vi "DataGridView Specific Column DEMO.vi"() -> ()   [LabVIEW 2011]
uses:
  System.Windows.Forms
panel:
  in  "stop":bool
  in  "DataGridView":refnum<k24>(container)
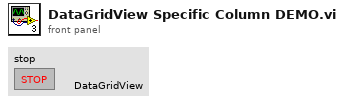
[diagram p1: front panel]
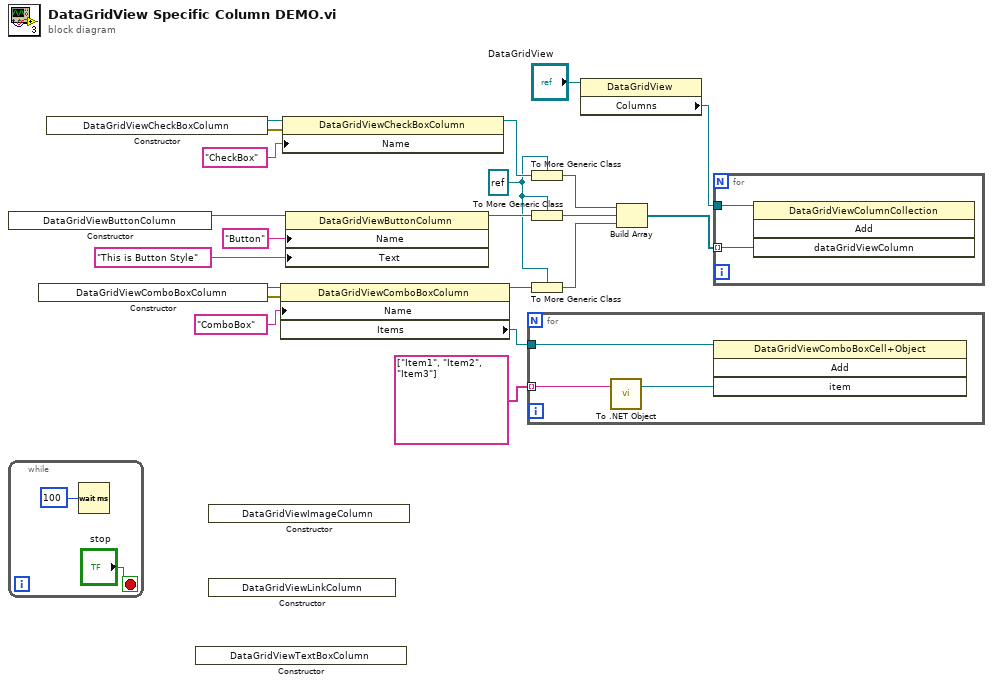
[diagram p0: block diagram]
diagram:
  w2 = refnum<k24> refnum ("dataGridViewColumn")
  n1 = constructor class="DataGridViewButtonColumn"() -> (reference out=w16:refnum<k24>)  [unwired: 3 in, 2 out]
  n2 = while {
    stop <- "stop" stop-if-true
    n3 = Wait (ms)(milliseconds to wait=u32 100) -> ()  [unwired: 1 out]
  }
  n4 = constructor class="DataGridViewComboBoxColumn"() -> (reference out=w7:refnum<k24>, error out=w8:errorcluster)  [unwired: 3 in, 1 out]
  n5 = constructor class="DataGridViewCheckBoxColumn"() -> (reference out=w20:refnum<k24>, error out=w19:errorcluster)  [unwired: 3 in, 1 out]
  n6 = constructor class="DataGridViewTextBoxColumn"() -> ()  [unwired: 3 in, 3 out]
  n7 = constructor class="DataGridViewImageColumn"() -> ()  [unwired: 3 in, 3 out]
  n8 = constructor class="DataGridViewLinkColumn"() -> ()  [unwired: 3 in, 3 out]
  n9 = property class="DataGridViewComboBoxColumn"(reference=w7, error in=w8, "Name"="ComboBox") -> (reference out=w3:refnum<k24>, "Items"=w4:refnum<k24>)  [unwired: 1 out]
  n10 = property class="DataGridViewCheckBoxColumn"(reference=w20, error in=w19, "Name"="CheckBox") -> (reference out=w13:refnum<k24>)  [unwired: 1 out]
  n11 = property class="DataGridViewButtonColumn"(reference=w16, "Name"="Button", "Text"="This is Button Style") -> (reference out=w12:refnum<k24>)  [unwired: 1 in, 1 out]
  n12 = for {
    tunnel: string[] ["Item1", "Item2", "Item3"] -> [w26] mode=indexing
    tunnel: w4 -> [w24]
    n13 = call <vilib>:"To .NET Object.vi"("anything"=w26) -> (".NET object"=w25:refnum<k24>)  [unwired: 1 in, 1 out]
    n14 = invoke class="DataGridViewComboBoxCell+Object" method="Add"(reference=w24, "item"=w25) -> ()  [unwired: 2 in, 4 out]
  }
  n15 = To More Generic Class(target class=w2, reference=w13) -> (generic class reference=w11:refnum<k24>)
  n16 = To More Generic Class(target class=w2, reference=w12) -> (generic class reference=w10:refnum<k24>)
  n17 = To More Generic Class(target class=w2, reference=w3) -> (generic class reference=w1:refnum<k24>)
  n18 = property class="DataGridView"(reference="DataGridView") -> ("Columns"=w17:refnum<k24>)  [unwired: 1 in, 2 out]
  n19 = Build Array(w11, w10, w1) -> (w9:refnum<k24>[])
  n20 = for {
    tunnel: w17 -> [w28]
    tunnel: w9 -> [w27] mode=indexing
    n21 = invoke class="DataGridViewColumnCollection" method="Add"(reference=w28, "dataGridViewColumn"=w27) -> ()  [unwired: 2 in, 4 out]
  }
